vi "Configure Generator Frequency.vi"(8 "error in (no error)":errorcluster, 10 "frequency, Hz":u32 format="%.0p", 11 "Arinst SSA-TG in":refnum<class "PL Arinst SSA-TG.lvclass">) -> (0 "error out":errorcluster, 3 "Arinst SSA-TG out":refnum<class "PL Arinst SSA-TG.lvclass">)   [LabVIEW 2015, in "PL Arinst SSA-TG.lvclass"]
doc: "Configures generator frequency."
uses:
  PL Arinst SSA-TG.lvclass
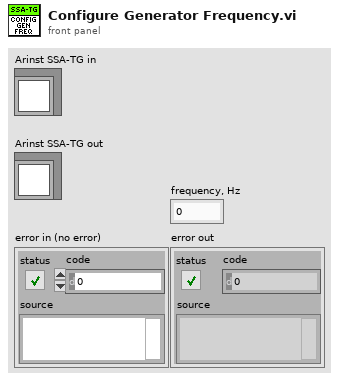
[diagram p1: front panel]
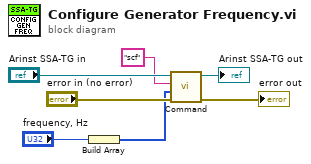
[diagram p0: block diagram]
diagram:
  n1 = Build Array("frequency, Hz") -> (w1:u32[])
  n2 = call "Command.vi"("error in (no error)"="error in (no error)", "arguments (none)"=w1, "command"="scf", "Arinst SSA-TG in"="Arinst SSA-TG in") -> ("error out"=→"error out":errorcluster, "Arinst SSA-TG out"=→"Arinst SSA-TG out":refnum<class "PL Arinst SSA-TG.lvclass">)  [unwired: 5 in, 1 out]
